vi "Lookup Object Hierarchy.vi"(8 "error in (no error)":errorcluster, 10 "LabVIEW Object":refnum<class>) -> (0 "error out":errorcluster, 1 "Library Versions":T1(array[cluster]), 2 "Private Data Clusters":variant[](array[variant]), 3 "Class Names":string[](array[string]))   [LabVIEW 2017, in "Composition.lvlib"]
doc: "Returns the private data clusters and version numbers for all classes in the object hierarchy in ascending order (most specific children first).\n\n<B>Note</B> This operation is very slow, which is why this VI holds a lookup table in memory to improve performance considerably."
uses:
  Composition.lvlib
  <vilib>/Utility/EditLVLibs/Edit LVLibs.lvlib
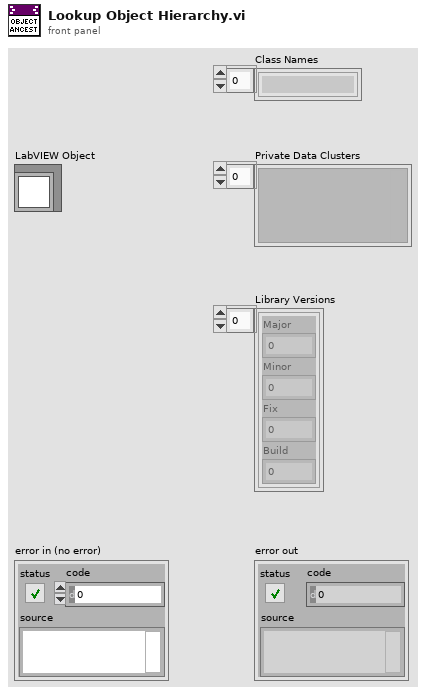
[diagram p1: front panel]
types:
  T1 = cluster{"Major":u16, "Minor":u16, "Fix":u16, "Build":u16}[]
  T2 = cluster{cluster{"Major":u16, "Minor":u16, "Fix":u16, "Build":u16}[]}[]
  T3 = typedef "Edit LVLibs.lvlib/LibVersion.ctl" = cluster{"Major":u16, "Minor":u16, "Fix":u16, "Build":u16}
  T4 = typedef "Edit LVLibs.lvlib/Mutation History.ctl" = T5[]
  T5 = typedef "Edit LVLibs.lvlib/Mutation Record.ctl" = cluster{"Library Version":T3, "Old Name Index":u8, "Class Default Data":variant, "Cluster Order Map":u32[], "Parent Name":string, "Parent Path":path, "LabVIEW Version":u32, "User Comments":string, "Mutation Flags":u8, "Parent Old Name Index":u8, "Parent Levels Added":u16, "Parent Levels Removed":u16}
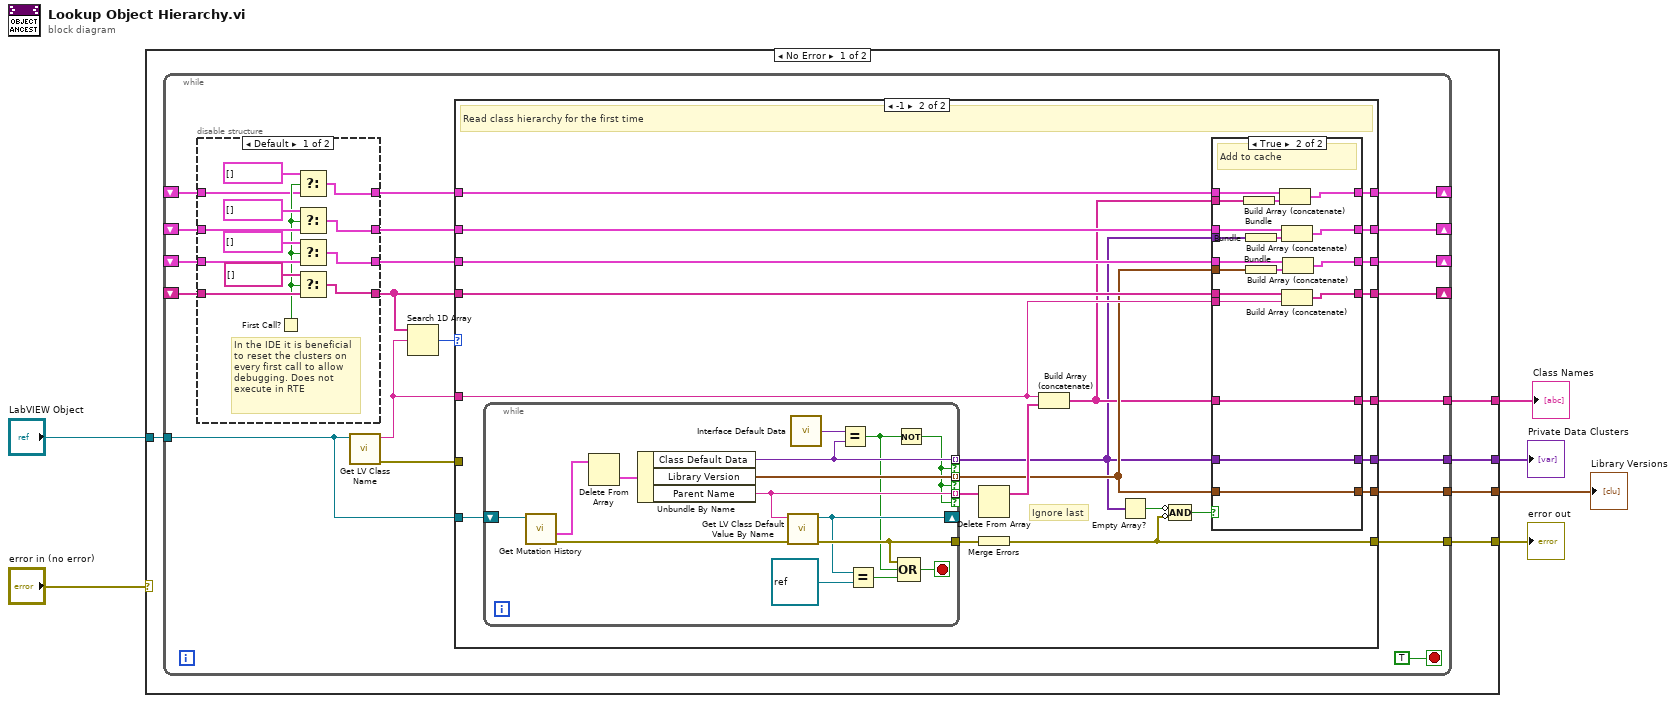
[diagram p0: block diagram]
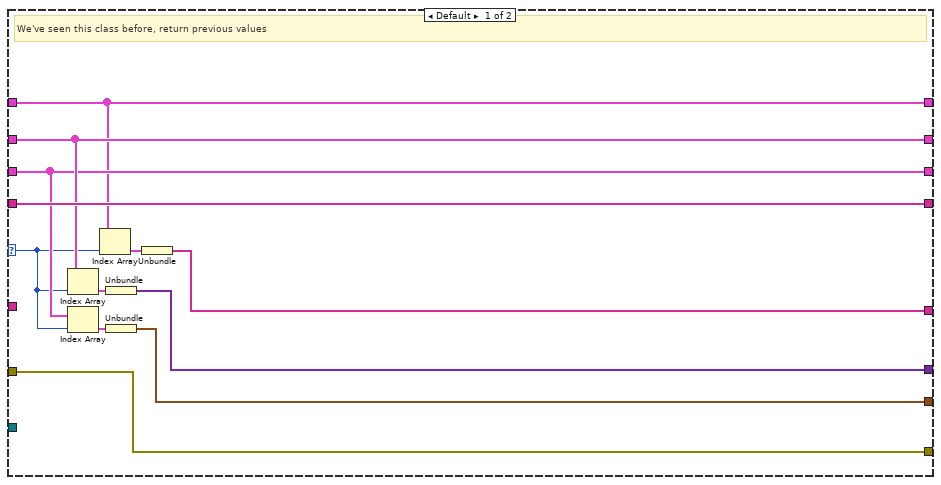
[diagram p2: hidden frame]
diagram:
  n1 = case shown="No Error" "error in (no error)" {
    selector: "error in (no error)" -> [_ w121]
    tunnel: "LabVIEW Object" -> [w11 _]
    tunnel: [w10 _] -> w5
    tunnel: [w9 w121] -> w3
    tunnel: [w8 _] -> w2
    tunnel: [w7 _] -> w1
    frame No Error {
      n2 = while {
        tunnel: w11 -> [w12]
        tunnel: [w32] -> w10
        tunnel: [w31] -> w9
        shift-right: [w29] -> _
        shift-left: _ -> [w23]
        shift-right: [w27] -> _
        shift-left: _ -> [w19]
        shift-right: [w26] -> _
        shift-left: _ -> [w21]
        tunnel: [w25] -> w8
        tunnel: [w16] -> w7
        shift-right: [w14] -> _
        shift-left: _ -> [w15]
        stop <- TRUE stop-if-true
        n3 = disable-structure shown="Default" {
          disable-tunnel: [w115 w120] -> w24
          disable-tunnel: w23 -> [w116 w120]
          disable-tunnel: [w111 w119] -> w22
          disable-tunnel: w21 -> [w114 w119]
          disable-tunnel: [w112 w118] -> w20
          disable-tunnel: w19 -> [w113 w118]
          disable-tunnel: w15 -> [w106 w117]
          disable-tunnel: [w105 w117] -> w13
          frame condition #0 (active) {
            # "In the IDE it is beneficial\nto reset the clusters on\nevery first call to allow\ndebugging. Does not\nexecute in RTE"
            n4 = First Call?() -> (First Call?: T/F=w107:bool)
            n5 = Select(t=cluster{string[]}[] [], s=w107, f=w106) -> (s? t:f=w105:cluster{string[]}[])
            n6 = Select(t=cluster{variant[]}[] [], s=w107, f=w116) -> (s? t:f=w115:cluster{variant[]}[])
            n7 = Select(t=T2 [], s=w107, f=w114) -> (s? t:f=w111:cluster{T3[]}[])
            n8 = Select(t=string[] [], s=w107, f=w113) -> (s? t:f=w112:string[])
          }
          frame condition #1 {
          }
        }
        n9 = call <vilib>:"Get LV Class Name.vi"("object"=w12) -> ("error out"=w17:errorcluster, "class name"=w18:string)  [unwired: 9 in]
        n10 = Search 1D Array(1D array=w20, element=w18) -> (index of element=w28:i32)  [unwired: 1 in]
        n11 = case shown="-1" w28 {
          selector: w28 -> [w35 _]
          tunnel: w18 -> [_ w56]
          tunnel: [w40 w49] -> w32
          tunnel: [w43 w53] -> w31
          tunnel: w24 -> [w42 w65]
          tunnel: w17 -> [w43 _]
          tunnel: [w42 w66] -> w29
          tunnel: w20 -> [w44 w64]
          tunnel: [w44 w63] -> w27
          tunnel: [w37 w50] -> w25
          tunnel: w22 -> [w38 w62]
          tunnel: [w38 w61] -> w26
          tunnel: [w33 w47] -> w16
          tunnel: [w34 w60] -> w14
          tunnel: w13 -> [w34 w59]
          tunnel: w12 -> [_ w57]
          frame Default {
            # "We've seen this class before, return previous values"
            n12 = Index Array(array=w42, index=w35) -> (element=w41:cluster{variant[]})
            n13 = Index Array(array=w38, index=w35) -> (element=w39:cluster{T3[]})
            n14 = Index Array(array=w34, index=w35) -> (element=w36:cluster{string[]})
            n15 = Unbundle(w41) -> (w40:variant[])
            n16 = Unbundle(w39) -> (w37:T3[])
            n17 = Unbundle(w36) -> (w33:string[])
          }
          frame -1 {
            # "Ignore last"
            # "Read class hierarchy for the first time"
            n18 = while {
              tunnel: [w72] -> w45 mode=indexing if=w69
              tunnel: [w76] -> w51 mode=indexing if=w69
              tunnel: [w77] -> w58
              shift-right: [w70] -> _
              shift-left: w57 -> [w79]
              tunnel: [w75] -> w55 mode=indexing if=w69
              stop <- w74 stop-if-true
              n19 = call <vilib>:"Get Mutation History.vi"("Input object"=w79) -> ("error out"=w78:errorcluster, "Mutation History"=w80:T4)  [unwired: 7 in]
              n20 = Delete From Array(array=w80) -> (deleted portion=w81:T5)  [unwired: 2 in, 1 out]
              n21 = Unbundle By Name(w81) -> ("Class Default Data"=w72:variant, "Library Version"=w76:T3, "Parent Name"=w75:string)
              n22 = call <vilib>:"Get LV Class Default Value By Name.vi"("error in (no error)"=w78, "class name"=w75) -> ("error out"=w77:errorcluster, "object"=w70:refnum<class>)  [unwired: 8 in]
              n23 = call "Interface Default Data.vi"() -> ("Interface Default Data"=w73:variant)  [unwired: 2 in]
              n24 = Equal?(x=w73, y=w72) -> (x = y?=w67:bool)
              n25 = Equal?(x=w70, y=refnum<class> refnum ("LabVIEW Object")) -> (x = y?=w68:bool)
              n26 = Not(x=w67) -> (.not. x?=w69:bool)
              n27 = Compound Arithmetic op=OR(w77, w67, w68) -> (w74:bool)
            }
            n28 = Delete From Array(array=w55) -> (array with subset deleted=w54:string[])  [unwired: 2 in, 1 out]
            n29 = Merge Errors(w58) -> (w53:errorcluster)
            n30 = Build Array (concatenate)(w56, w54) -> (w48:string[])
            n31 = Empty Array?(array=w45) -> (empty?=w46:bool)
            n32 = Compound Arithmetic op=AND(invert w46, invert w53) -> (w52:bool)
            n33 = case shown="True" w52 {
              tunnel: [w84 w103] -> w66
              tunnel: w65 -> [w84 w102]
              tunnel: w64 -> [w82 w101]
              tunnel: w56 -> [_ w100]
              tunnel: [w82 w99] -> w63
              tunnel: w45 -> [_ w98]
              tunnel: w62 -> [w83 w96]
              tunnel: [w83 w95] -> w61
              tunnel: w51 -> [_ w94]
              tunnel: [w85 w91] -> w60
              tunnel: w48 -> [_ w90]
              tunnel: w59 -> [w85 w89]
              tunnel: w51 -> [_ w88]
              tunnel: [_ w88] -> w50
              tunnel: w45 -> [_ w87]
              tunnel: [_ w87] -> w49
              tunnel: w48 -> [_ w86]
              tunnel: [_ w86] -> w47
              frame False {
                # "Don't cache"
              }
              frame True {
                # "Add to cache"
                n34 = Bundle(w90) -> (w92:cluster{string[]})  [unwired: 1 in]
                n35 = Bundle(w98) -> (w97:cluster{variant[]})  [unwired: 1 in]
                n36 = Bundle(w94) -> (w93:cluster{T3[]})  [unwired: 1 in]
                n37 = Build Array (concatenate)(w89, w92) -> (w91:cluster{string[]}[])
                n38 = Build Array (concatenate)(w102, w97) -> (w103:cluster{variant[]}[])
                n39 = Build Array (concatenate)(w101, w100) -> (w99:string[])
                n40 = Build Array (concatenate)(w96, w93) -> (w95:cluster{T3[]}[])
              }
            }
          }
        }
      }
    }
    frame Error {
    }
  }
  "Private Data Clusters" <- w5
  "error out" <- w3
  "Library Versions" <- w2
  "Class Names" <- w1
